vi "AddFrontPanelControls.vi"(5 "Open Front Panel":bool, 6 "write?":bool, 7 "Control Properties":T1[](array[typedef])=[{"label"="tag bus in ", "terminal index"=11, "indicator"=FALSE, "location"={"Horizontal"=0, "Vertical"=0}}, {"label"="tag bus out", "terminal index"=3, "indicator"=TRUE, "location"={"Horizontal"=600, "Vertical"=0}}, {"label"="cluster", "terminal index"=10, "indicator"=FALSE, "location"={"Horizontal"=200, "Vertical"=0}}, {"label"="index cluster", "terminal index"=2, "indicator"=FALSE, "location"={"Horizontal"=400, "Vertical"=0}}, {"label"="error in", "terminal index"=8, "indicator"=FALSE, "location"={"Horizontal"=0, "Vertical"=400}}, {"label"="error out", "terminal index"=0, "indicator"=TRUE, "location"={"Horizontal"=600, "Vertical"=400}}], 8 "error in":errorcluster, 11 "State":T3={"paths"={"index cluster path"=path "C:/Users/bcelis.AMER/Documents/TBDCore/source/Utilities/Cluster to Tag Bus Scripts/Controls/IndexCluster.ctl", "cluster path"=path "C:/Users/bcelis.AMER/Documents/TBDCore/source/Utilities/Cluster to Tag Bus Scripts/Controls/SampleControl.ctl", "cluster to tag bus VI path"=path "C:/Users/bcelis.AMER/Documents/TBDCore/source/Utilities/Cluster to Tag Bus Scripts/ClustertoTagbus.vi", " tag bus to cluster VI path"=path ""}, "write VI ref"=refnum, "read VI ref"=refnum, "base cluster"=variant}) -> (0 "error out":errorcluster, 2 "Terminal References":T5, 3 "State out":T3={"paths"={"index cluster path"=path "C:/Users/bcelis.AMER/Documents/TBDCore/source/Utilities/Cluster to Tag Bus Scripts/Controls/IndexCluster.ctl", "cluster path"=path "C:/Users/bcelis.AMER/Documents/TBDCore/source/Utilities/Cluster to Tag Bus Scripts/Controls/SampleControl.ctl", "cluster to tag bus VI path"=path "C:/Users/bcelis.AMER/Documents/TBDCore/source/Utilities/Cluster to Tag Bus Scripts/ClustertoTagbus.vi", " tag bus to cluster VI path"=path ""}, "write VI ref"=refnum, "read VI ref"=refnum, "base cluster"=variant})   [LabVIEW 2013]
uses:
  Controls/TerminalReferences.ctl
  Controls/StateCluster.ctl
  Controls/PathsCluster.ctl
  Controls/ControlsProperties.ctl
  <vilib>/Utility/miscctls.llb/LVPointTypeDef.ctl
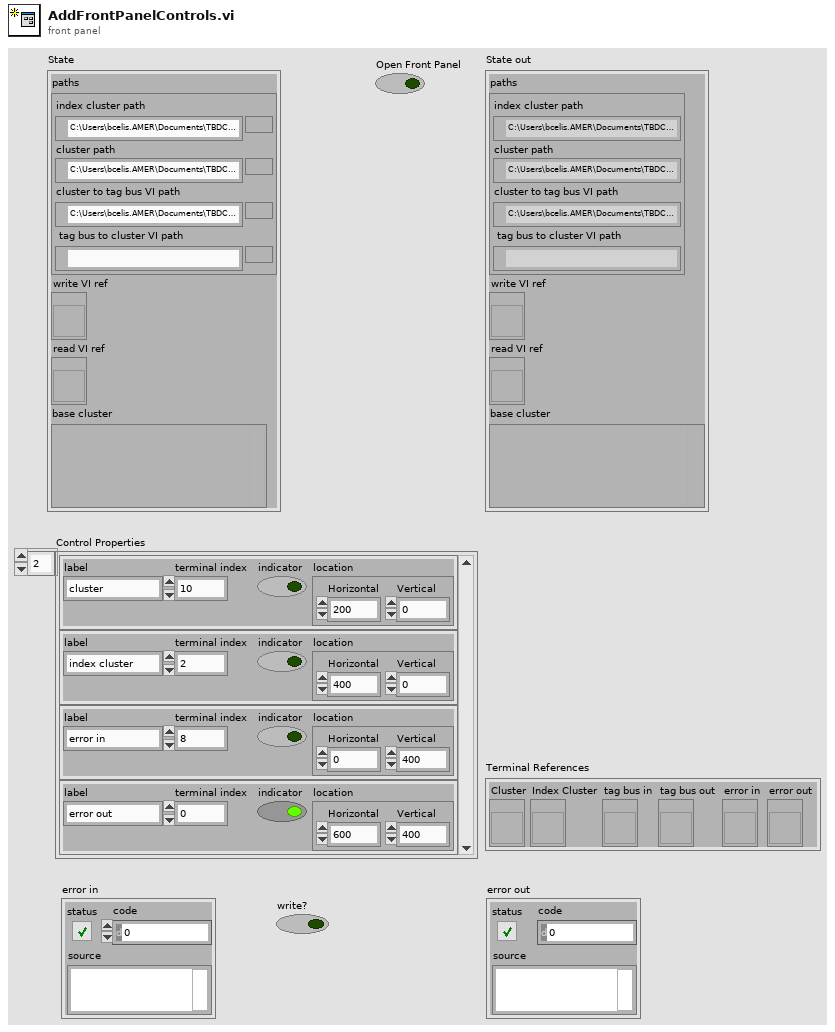
[diagram p1: front panel]
types:
  T1 = typedef "ControlsProperties.ctl" = cluster{"label":string, "terminal index":u32, "indicator":bool, "location":T2}
  T2 = typedef "LVPointTypeDef.ctl" = cluster{"Horizontal":i16, "Vertical":i16}
  T3 = typedef "StateCluster.ctl" = cluster{"paths":T4, "write VI ref":refnum<vi>, "read VI ref":refnum<vi>, "base cluster":variant}
  T4 = typedef "PathsCluster.ctl" = cluster{"index cluster path":path, "cluster path":path, "cluster to tag bus VI path":path, " tag bus to cluster VI path":path}
  T5 = typedef "TerminalReferences.ctl" = cluster{"Cluster":refnum<vi>, "Index Cluster":refnum<vi>, "tag bus in":refnum<vi>, "tag bus out":refnum<vi>, "error in ":refnum<vi>, "error out":refnum<vi>}
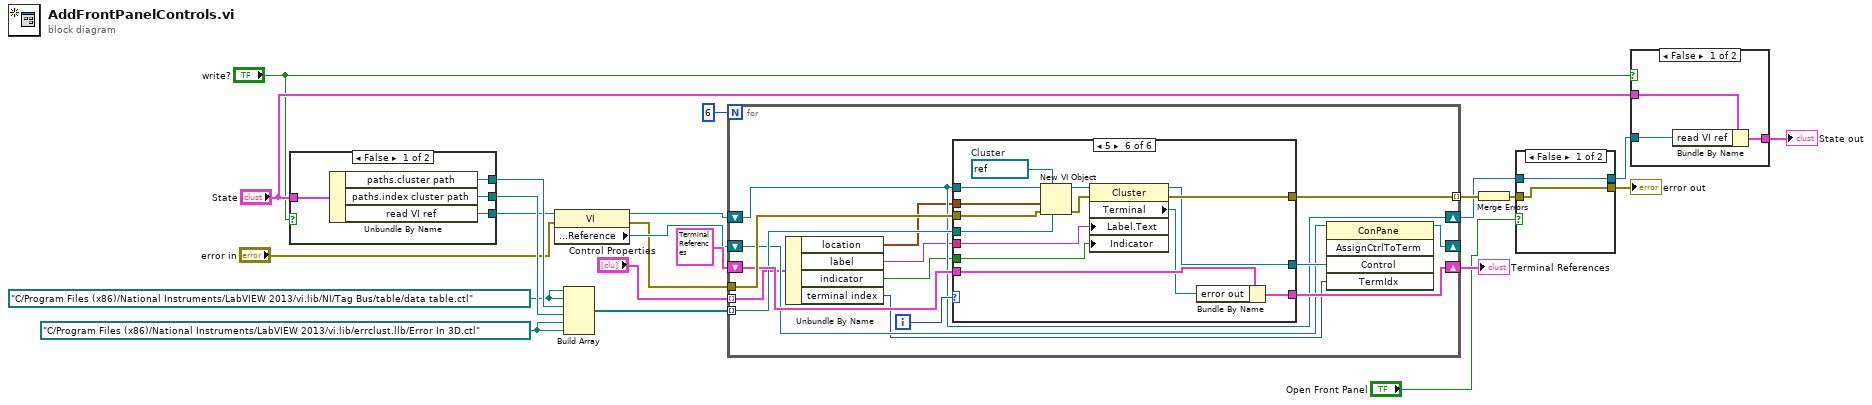
[diagram p0: block diagram]
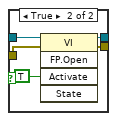
[diagram p2: hidden frame]
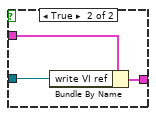
[diagram p3: hidden frame]
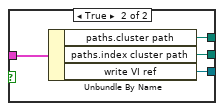
[diagram p4: hidden frame]
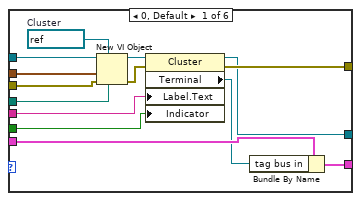
[diagram p5: hidden frame]
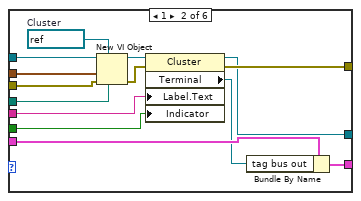
[diagram p6: hidden frame]
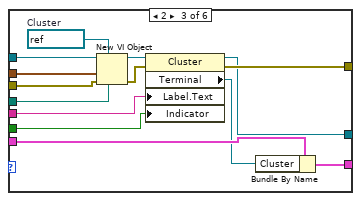
[diagram p7: hidden frame]
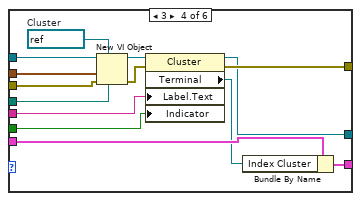
[diagram p8: hidden frame]
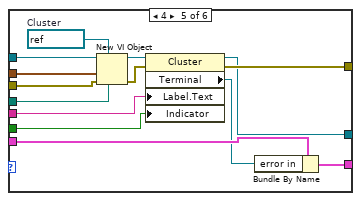
[diagram p9: hidden frame]
diagram:
  w15 = path "C:/Program Files (x86)/National Instruments/LabVIEW 2013/vi.lib/NI/Tag Bus/table/data table.ctl" ("element")
  w19 = path "C:/Program Files (x86)/National Instruments/LabVIEW 2013/vi.lib/errclust.llb/Error In 3D.ctl" ("element")
  n1 = case shown="False" "write?" {
    tunnel: [w27 w31] -> w21
    tunnel: [w26 w30] -> w18
    tunnel: "State" -> [w25 w29]
    tunnel: [w24 w28] -> w11
    frame False {
      n2 = Unbundle By Name(w25) -> ("paths.cluster path"=w27:path, "paths.index cluster path"=w26:path, "read VI ref"=w24:refnum<vi>)
    }
    frame True {
      n3 = Unbundle By Name(w29) -> ("paths.cluster path"=w31:path, "paths.index cluster path"=w30:path, "write VI ref"=w28:refnum<vi>)
    }
  }
  n4 = property class="VI"(reference=w11, error in="error in") -> (reference out=w14:refnum<vi>, error out=w2:errorcluster, "Connector Pane:Reference"=w13:refnum<vi>)
  n5 = Build Array(w15, w15, w21, w18, w19, w19) -> (w20:path[])
  n6 = for {
    N: 6 -> [_]
    tunnel: w2 -> [w46]
    tunnel: w20 -> [w43] mode=indexing
    shift-right: [w44] -> w22
    shift-left: T5 {"Cluster"=refnum, "Index Cluster"=refnum, "tag bus in"=refnum, "tag bus out"=refnum, "error in "=refnum, "error out"=refnum} ("Terminal References") -> [w45]
    tunnel: [w41] -> w16 mode=indexing
    shift-right: [w38] -> _
    shift-left: w13 -> [w39]
    shift-right: [w37] -> w7
    shift-left: w14 -> [w37]
    tunnel: "Control Properties" -> [w36] mode=indexing
    i -> [w42]
    n7 = Unbundle By Name(w36) -> ("location"=w34:T2, "label"=w35:string, "indicator"=w33:bool, "terminal index"=w32:u32)
    n8 = case shown="5" w42 {
      tunnel: w46 -> [w59 w73 w87 w101 w115 w129]
      tunnel: w45 -> [w58 w72 w86 w100 w114 w128]
      tunnel: [w57 w71 w85 w99 w113 w127] -> w44
      tunnel: w43 -> [w55 w69 w83 w97 w111 w125]
      tunnel: w34 -> [w53 w67 w81 w95 w109 w123]
      tunnel: [w52 w66 w80 w94 w108 w122] -> w41
      tunnel: w37 -> [w51 w65 w79 w93 w107 w120]
      tunnel: w35 -> [w48 w62 w76 w90 w104 w121]
      tunnel: [w49 w63 w77 w91 w105 w118] -> w40
      tunnel: w33 -> [w47 w61 w75 w89 w103 w117]
      frame 0, Default {
        w60 = refnum<vi> refnum  # Cluster
        n9 = New VI Object(vi object class=w60, owner refnum=w51, position/next to=w53, 6:w55, 8:w59) -> (object refnum=w50:refnum<vi>, 0:w54:errorcluster)  [unwired: 3 in]
        n10 = property on="Property Node" class="Cluster"(reference=w50, error in=w54, "Label.Text"=w48, "Indicator"=w47) -> (reference out=w49:refnum<vi>, error out=w52:errorcluster, "Terminal"=w56:refnum<vi>)
        n11 = Bundle By Name(cluster=w58, "tag bus in"=w56) -> (w57:T5)
      }
      frame 1 {
        w74 = refnum<vi> refnum  # Cluster
        n12 = New VI Object(vi object class=w74, owner refnum=w65, position/next to=w67, 6:w69, 8:w73) -> (object refnum=w64:refnum<vi>, 0:w68:errorcluster)  [unwired: 3 in]
        n13 = property on="Property Node" class="Cluster"(reference=w64, error in=w68, "Label.Text"=w62, "Indicator"=w61) -> (reference out=w63:refnum<vi>, error out=w66:errorcluster, "Terminal"=w70:refnum<vi>)
        n14 = Bundle By Name(cluster=w72, "tag bus out"=w70) -> (w71:T5)
      }
      frame 2 {
        w88 = refnum<vi> refnum  # Cluster
        n15 = New VI Object(vi object class=w88, owner refnum=w79, position/next to=w81, 6:w83, 8:w87) -> (object refnum=w78:refnum<vi>, 0:w82:errorcluster)  [unwired: 3 in]
        n16 = property on="Property Node" class="Cluster"(reference=w78, error in=w82, "Label.Text"=w76, "Indicator"=w75) -> (reference out=w77:refnum<vi>, error out=w80:errorcluster, "Terminal"=w84:refnum<vi>)
        n17 = Bundle By Name(cluster=w86, "Cluster"=w84) -> (w85:T5)
      }
      frame 3 {
        w102 = refnum<vi> refnum  # Cluster
        n18 = New VI Object(vi object class=w102, owner refnum=w93, position/next to=w95, 6:w97, 8:w101) -> (object refnum=w92:refnum<vi>, 0:w96:errorcluster)  [unwired: 3 in]
        n19 = property on="Property Node" class="Cluster"(reference=w92, error in=w96, "Label.Text"=w90, "Indicator"=w89) -> (reference out=w91:refnum<vi>, error out=w94:errorcluster, "Terminal"=w98:refnum<vi>)
        n20 = Bundle By Name(cluster=w100, "Index Cluster"=w98) -> (w99:T5)
      }
      frame 4 {
        w116 = refnum<vi> refnum  # Cluster
        n21 = New VI Object(vi object class=w116, owner refnum=w107, position/next to=w109, 6:w111, 8:w115) -> (object refnum=w106:refnum<vi>, 0:w110:errorcluster)  [unwired: 3 in]
        n22 = property on="Property Node" class="Cluster"(reference=w106, error in=w110, "Label.Text"=w104, "Indicator"=w103) -> (reference out=w105:refnum<vi>, error out=w108:errorcluster, "Terminal"=w112:refnum<vi>)
        n23 = Bundle By Name(cluster=w114, "error in"=w112) -> (w113:T5)
      }
      frame 5 {
        w130 = refnum<vi> refnum  # Cluster
        n24 = New VI Object(vi object class=w130, owner refnum=w120, position/next to=w123, 6:w125, 8:w129) -> (object refnum=w119:refnum<vi>, 0:w124:errorcluster)  [unwired: 3 in]
        n25 = property on="Property Node" class="Cluster"(reference=w119, error in=w124, "Label.Text"=w121, "Indicator"=w117) -> (reference out=w118:refnum<vi>, error out=w122:errorcluster, "Terminal"=w126:refnum<vi>)
        n26 = Bundle By Name(cluster=w128, "error out"=w126) -> (w127:T5)
      }
    }
    n27 = invoke class="ConPane" method="AssignCtrlToTerm"(reference=w39, "Control"=w40, "TermIdx"=w32) -> (reference out=w38:refnum<vi>)  [unwired: 2 in, 4 out]
  }
  "Terminal References" <- w22
  n28 = Merge Errors(w16) -> (w5:errorcluster)
  n29 = case shown="False" "Open Front Panel" {
    tunnel: w7 -> [w132 w136]
    tunnel: [w132 w135] -> w6
    tunnel: w5 -> [w131 w134]
    tunnel: [w131 w133] -> w4
    frame False {
    }
    frame True {
      n30 = invoke class="VI" method="FP.Open"(reference=w136, error in=w134, "Activate"=TRUE ("Activate?")) -> (reference out=w135:refnum<vi>, error out=w133:errorcluster)  [unwired: 2 in, 3 out]
    }
  }
  "error out" <- w4
  n31 = case shown="False" "write?" {
    tunnel: "State" -> [w140 w143]
    tunnel: w6 -> [w139 w142]
    tunnel: [w138 w141] -> w9
    frame False {
      n32 = Bundle By Name(cluster=w140, "read VI ref"=w139) -> (w138:T3)
    }
    frame True {
      n33 = Bundle By Name(cluster=w143, "write VI ref"=w142) -> (w141:T3)
    }
  }
  "State out" <- w9
